vi "sequenc buffer.vi"() -> ()   [LabVIEW 2013]
panel:
  in  "stop":bool
  in  "Number of Images":u32=5
  out "All Images Out":T1[](array[plugin-control])
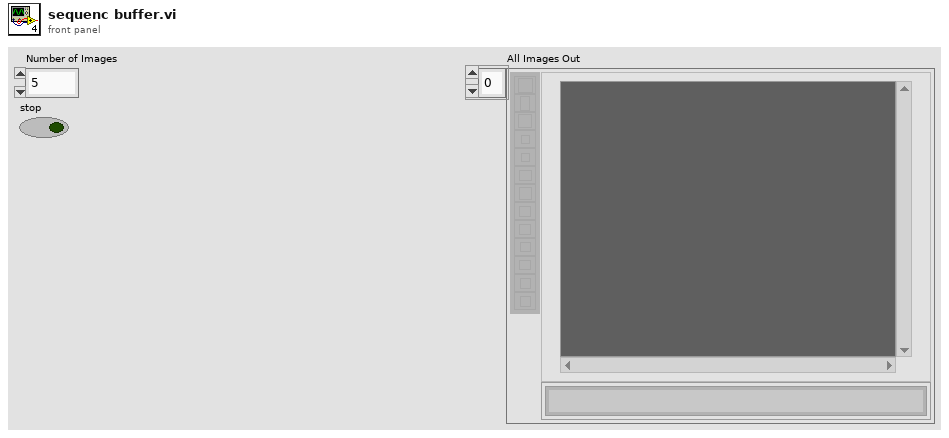
[diagram p1: front panel]
types:
  T1 = typedef "IMAQ Image.ctl" = refnum<image>
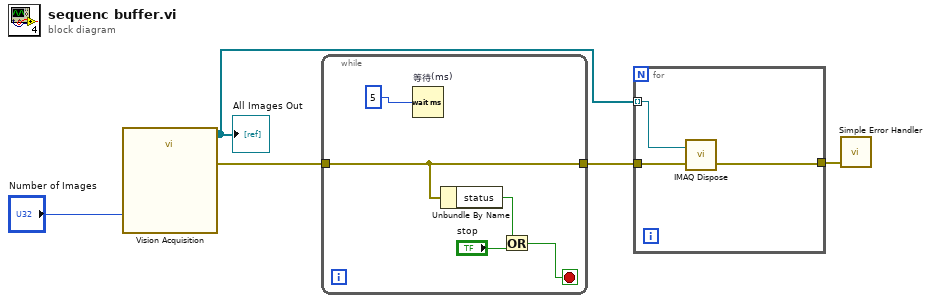
[diagram p0: block diagram]
diagram:
  n1 = call "Vision Acquisition"("Number of Images"="Number of Images") -> ("All Images Out"=w2:T1[], "error out"=w4:errorcluster)  [unwired: 25 in]
  "All Images Out" <- w2
  n2 = while {
    tunnel: w4 -> [w9]
    tunnel: [w9] -> w3
    stop <- w7 stop-if-true
    n3 = Wait (ms) "等待(ms)"(milliseconds to wait=u32 5 ("毫秒计时值")) -> ()  [unwired: 1 out]
    n4 = Unbundle By Name(w9) -> ("status"=w8:bool)
    n5 = Or(x=w8, y="stop") -> (x .or. y?=w7:bool)
  }
  n6 = for {
    tunnel: w3 -> [w13]
    tunnel: w2 -> [w12] mode=indexing
    tunnel: [w11] -> w1
    n7 = call "IMAQ Dispose"("Image"=w12, "error in (no error)"=w13) -> ("error out"=w11:errorcluster)  [unwired: 4 in]
  }
  n8 = call <vilib>:"Simple Error Handler.vi"("error in (no error)"=w1) -> ()  [unwired: 4 in, 5 out]
